vi "Write Serial Data.vi"(8 "error in":errorcluster, 10 "CRD Data In":refnum<class "CRDS Data.lvclass">, 11 "File Obs in":refnum<class "CRD File Obs.lvclass">) -> (0 "error out":errorcluster, 2 "CRD Data Out":refnum<class "CRDS Data.lvclass">, 3 "File Obs Out":refnum<class "CRD File Obs.lvclass">)   [LabVIEW 2015, in "CRD File Obs.lvclass"]
uses:
  CRD File Obs.lvclass
  Data/Main/CRDS Data.lvclass
  Instruments/AOP/CRDS/Data/cCRDS Data.lvclass
  Devices/Alicat/Session Based/Data/Alicat Data.lvclass
  Instruments/AOP/CRDS/Data/cCRDS Data.lvclass/cCRDS Data.ctl
  File IO/Class/File Observer.lvclass/File Observer.ctl
  Data/Main/crd_data_enum.ctl
  Instruments/AOP/CRDS/Data/Read Serial Data.vi
  File IO/Class/Read File Ref.vi
  Data/Data.lvclass
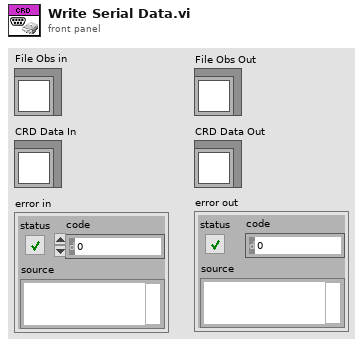
[diagram p1: front panel]
types:
  T1 = enum16{"big-endian, network order", "native, host order", "little-endian"}
  T2 = typedef "crd_data_enum.ctl" = enum8{"Time", "RHw", "TRH", "P", "Tmean", "RHsense", "TQ", "PQ", "Q", "Q0", "Qcal", "Qset", "extDilFac", "taucorr", "tau0corr", "stdevtau", "ext", "extCorr", "etau", "tau", "tau0", "Purge_Data", "NoData", "reserved", "Ttec", "Ang Exp", "Gamma", "filter", "fOverride", "notes", "max amp", "Tthermistor", "RhdilFac", "Psense", "TRHsense_bank", "RHsense_bank", "MFC_Data", "Thum", "ThumSP", "O3 Flow", "Pinlet Flow", "CLAP Flow", "O3 Add Valve", "O2 Valve", "O3 Cal"}
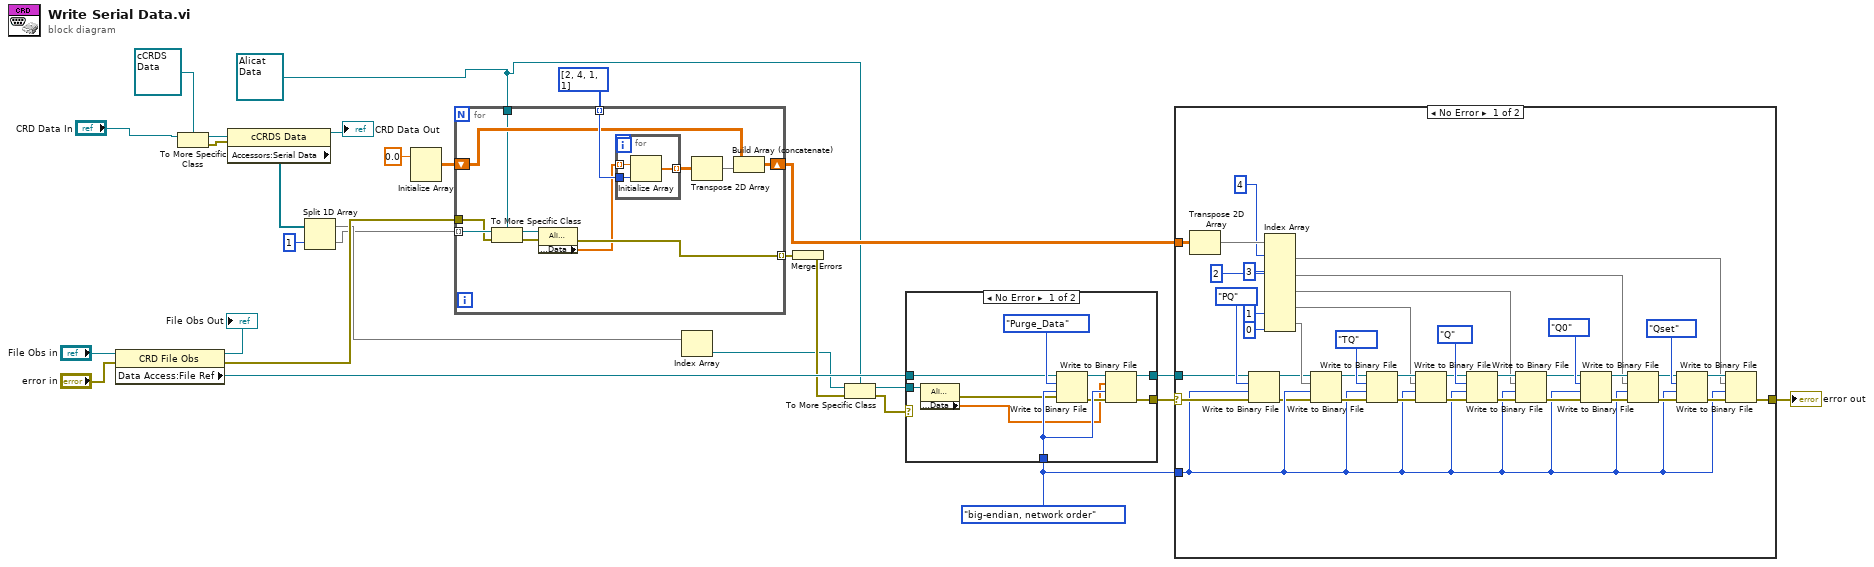
[diagram p0: block diagram]
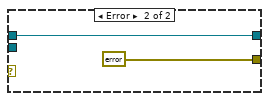
[diagram p2: hidden frame]
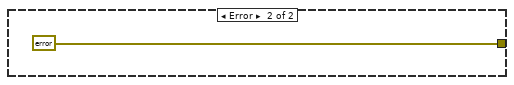
[diagram p3: hidden frame]
diagram:
  w1 = refnum<class "Alicat Data.lvclass"> refnum ("Alicat Data")
  w27 = T1."big-endian, network order" ("byte order (0:big-endian, network order)")
  n1 = property class="CRD File Obs"(reference="File Obs in", error in="error in") -> (reference out=→"File Obs Out":refnum<class "CRD File Obs.lvclass">, error out=w15:errorcluster, "Data Access:File Ref"=w21:refnum<file>)
  n2 = To More Specific Class(target class=refnum<class "cCRDS Data.lvclass"> refnum ("cCRDS Data"), reference="CRD Data In") -> (specific class reference=w12:refnum<class "cCRDS Data.lvclass">, error out=w11:errorcluster)  [unwired: 1 in]
  n3 = property class="cCRDS Data"(reference=w12, error in=w11) -> (reference out=→"CRD Data Out":refnum<class "cCRDS Data.lvclass">, "Accessors:Serial Data"=w9:refnum<class "Data.lvclass">[])  [unwired: 1 out]
  n4 = Split 1D Array(array=w9, index=1) -> (first subarray=w5:refnum<class "Data.lvclass">[], second subarray=w3:refnum<class "Data.lvclass">[])
  n5 = Initialize Array(sgl 0.0 ("element")) -> (w26:sgl[][])  [unwired: 2 in]
  n6 = for {
    tunnel: w3 -> [w40] mode=indexing
    tunnel: i32[] [2, 4, 1, 1] -> [w39] mode=indexing
    shift-right: [w35] -> w2
    shift-left: w26 -> [w36]
    tunnel: [w30] -> w28 mode=indexing
    tunnel: w15 -> [w34]
    tunnel: w1 -> [w33]
    n7 = To More Specific Class(target class=w33, reference=w40, error in=w34) -> (specific class reference=w32:refnum<class "Alicat Data.lvclass">, error out=w31:errorcluster)
    n8 = property class="Alicat Data"(reference=w32, error in=w31) -> (error out=w30:errorcluster, "Accessors:Data"=w29:sgl[])  [unwired: 1 out]
    n9 = for {
      tunnel: w29 -> [w43] mode=indexing
      tunnel: w39 -> [w42]
      tunnel: [w41] -> w38 mode=indexing
      n10 = Initialize Array(w43, w42) -> (w41:sgl[])
    }
    n11 = Transpose 2D Array(2D array=w38) -> (transposed array=w37:sgl[][])
    n12 = Build Array (concatenate)(w36, w37) -> (w35:sgl[][])
  }
  n13 = Index Array(array=w5) -> (element=w4:refnum<class "Data.lvclass">)  [unwired: 1 in]
  n14 = Merge Errors(w28) -> (w18:errorcluster)
  n15 = To More Specific Class(target class=w1, reference=w4, error in=w18) -> (specific class reference=w6:refnum<class "Alicat Data.lvclass">, error out=w7:errorcluster)
  n16 = case shown="No Error" w7 {
    tunnel: w6 -> [w48 _]
    tunnel: w27 -> [w53 _]
    tunnel: [w45 errorcluster {"status"=FALSE, "code"=0, "source"=""} ("error out")] -> w16
    tunnel: [w46 w54] -> w22
    tunnel: w21 -> [w49 w54]
    frame No Error {
      n17 = property class="Alicat Data"(reference=w48) -> (error out=w47:errorcluster, "Accessors:Data"=w44:sgl[])  [unwired: 1 in, 1 out]
      n18 = Write to Binary File(file (use dialog)=w49, data=crd_data_enum."Purge_Data" ("CRD_Data_Enum"), error in=w47, 9:w53) -> (refnum out=w52:refnum<file>, error out=w50:errorcluster)  [unwired: 2 in, 1 out]
      n19 = Write to Binary File(file (use dialog)=w52, data=w44, error in=w50, 9:w53) -> (refnum out=w46:refnum<file>, error out=w45:errorcluster)  [unwired: 2 in, 1 out]
    }
    frame Error {
    }
  }
  n20 = case shown="No Error" w16 {
    selector: w16 -> [w64 _]
    tunnel: w27 -> [w63 _]
    tunnel: [w94 errorcluster {"status"=FALSE, "code"=0, "source"=""} ("error out")] -> w17
    tunnel: w22 -> [w65 _]
    tunnel: w2 -> [w68 _]
    frame No Error {
      n21 = Transpose 2D Array(2D array=w68) -> (transposed array=w67:sgl[][])
      n22 = Write to Binary File(file (use dialog)=w65, data=crd_data_enum."PQ" ("CRD_Data_Enum"), error in=w64, 9:w63) -> (refnum out=w62:refnum<file>, error out=w61:errorcluster)  [unwired: 2 in, 1 out]
      n23 = Index Array(array=w67, index (row) #1=4 ("index (row)"), index (row) #2=3 ("index (row)"), index (row) #3=2 ("index (row)"), index (row) #4=1 ("index (row)"), index (row) #5=0 ("index (row)")) -> (element #1=w73:sgl[], element #2=w72:sgl[], element #3=w71:sgl[], element #4=w70:sgl[], element #5=w69:sgl[])  [unwired: 5 in]
      n24 = Write to Binary File(file (use dialog)=w62, data=w69, error in=w61, 9:w63) -> (refnum out=w90:refnum<file>, error out=w89:errorcluster)  [unwired: 2 in, 1 out]
      n25 = Write to Binary File(file (use dialog)=w90, data=crd_data_enum."TQ" ("CRD_Data_Enum"), error in=w89, 9:w63) -> (refnum out=w93:refnum<file>, error out=w92:errorcluster)  [unwired: 2 in, 1 out]
      n26 = Write to Binary File(file (use dialog)=w93, data=w70, error in=w92, 9:w63) -> (refnum out=w85:refnum<file>, error out=w84:errorcluster)  [unwired: 2 in, 1 out]
      n27 = Write to Binary File(file (use dialog)=w85, data=crd_data_enum."Q" ("CRD_Data_Enum"), error in=w84, 9:w63) -> (refnum out=w87:refnum<file>, error out=w88:errorcluster)  [unwired: 2 in, 1 out]
      n28 = Write to Binary File(file (use dialog)=w87, data=w71, error in=w88, 9:w63) -> (refnum out=w80:refnum<file>, error out=w79:errorcluster)  [unwired: 2 in, 1 out]
      n29 = Write to Binary File(file (use dialog)=w80, data=crd_data_enum."Q0" ("CRD_Data_Enum"), error in=w79, 9:w63) -> (refnum out=w83:refnum<file>, error out=w82:errorcluster)  [unwired: 2 in, 1 out]
      n30 = Write to Binary File(file (use dialog)=w83, data=w72, error in=w82, 9:w63) -> (refnum out=w75:refnum<file>, error out=w74:errorcluster)  [unwired: 2 in, 1 out]
      n31 = Write to Binary File(file (use dialog)=w75, data=crd_data_enum."Qset" ("CRD_Data_Enum"), error in=w74, 9:w63) -> (refnum out=w77:refnum<file>, error out=w78:errorcluster)  [unwired: 2 in, 1 out]
      n32 = Write to Binary File(file (use dialog)=w77, data=w73, error in=w78, 9:w63) -> (error out=w94:errorcluster)  [unwired: 2 in, 2 out]
    }
    frame Error {
    }
  }
  "error out" <- w17
